vi "Total channel count.vi"(11 "Acquisition config":T1(array[cluster])=[{"Channel status"=0.0, "Channel count"=0, "Module active"=FALSE}, {"Channel status"=0.0, "Channel count"=0, "Module active"=FALSE}, {"Channel status"=0.0, "Channel count"=0, "Module active"=FALSE}, {"Channel status"=0.0, "Channel count"=0, "Module active"=FALSE}, {"Channel status"=0.0, "Channel count"=0, "Module active"=FALSE}, {"Channel status"=0.0, "Channel count"=0, "Module active"=FALSE}, {"Channel status"=0.0, "Channel count"=0, "Module active"=FALSE}, {"Channel status"=0.0, "Channel count"=0, "Module active"=FALSE}]) -> (3 "Total channels":u8)   [LabVIEW 2018]
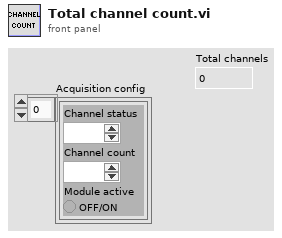
[diagram p1: front panel]
types:
  T1 = cluster{"Channel status":fxp<+,32,32>, "Channel count":u8, "Module active":bool}[]
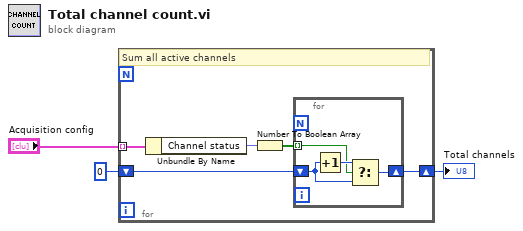
[diagram p0: block diagram]
diagram:
  n1 = for {
    tunnel: "Acquisition config" -> [w8] mode=indexing
    shift-right: [w4] -> w1
    shift-left: u8 0 -> [w5]
    # "Sum all active channels"
    n2 = Unbundle By Name(w8) -> ("Channel status"=w7:fxp<+,32,32>)
    n3 = Number To Boolean Array(number=w7) -> (Boolean array=w6:bool[])
    n4 = for {
      tunnel: w6 -> [w11] mode=indexing
      shift-right: [w9] -> w4
      shift-left: w5 -> [w10]
      n5 = Increment(x=w10) -> (x+1=w12:u8)
      n6 = Select(t=w12, s=w11, f=w10) -> (s? t:f=w9:u8)
    }
  }
  "Total channels" <- w1
